vi "Get Feature Names.vi"(8 "error in (no error)":errorcluster caption="entrée d'erreur (pas d'erreur)", 9 "doc":string, 10 "X":string[][](array[string]), 11 "TfidfVectorizer.lvclass":refnum<class "TfidfVectorizer.lvclass">) -> (0 "error out":errorcluster caption="sortie d'erreur", 2 "Data":T1, 3 "TfidfVectorizer.lvclass":refnum<class "TfidfVectorizer.lvclass">)   [LabVIEW 2020, in "TfidfVectorizer.lvclass"]
doc: "Array mapping from feature integer indices to feature name.\n\nReturns : \n\n- feature_names : list\nA list of feature names."
uses:
  TfidfVectorizer.lvclass
  TfidfVectorizer.lvclass/TfidfVectorizer.ctl
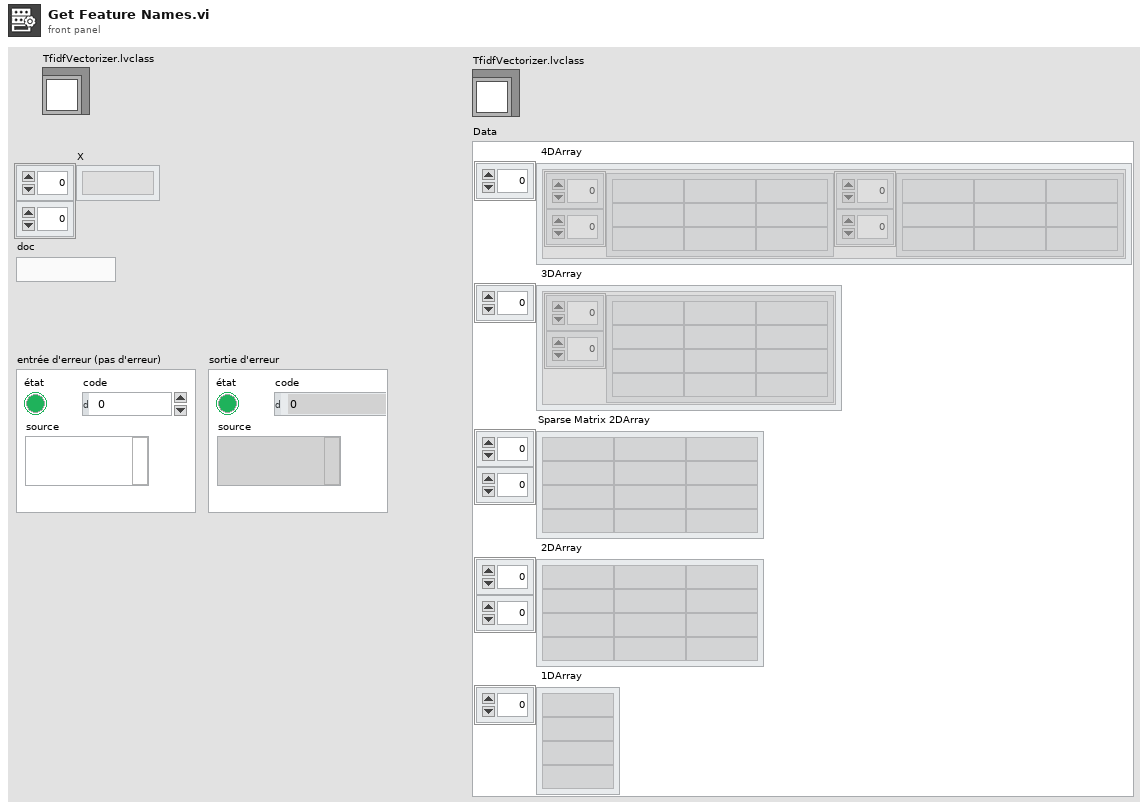
[diagram p1: front panel]
types:
  T1 = cluster{" 4DArray":cluster{"1":string[][], "2":string[][]}[], " 3DArray":cluster{"Tableau":string[][]}[], "Sparse Matrix 2DArray":string[][], " 2DArray":string[][], " 1DArray":string[]}
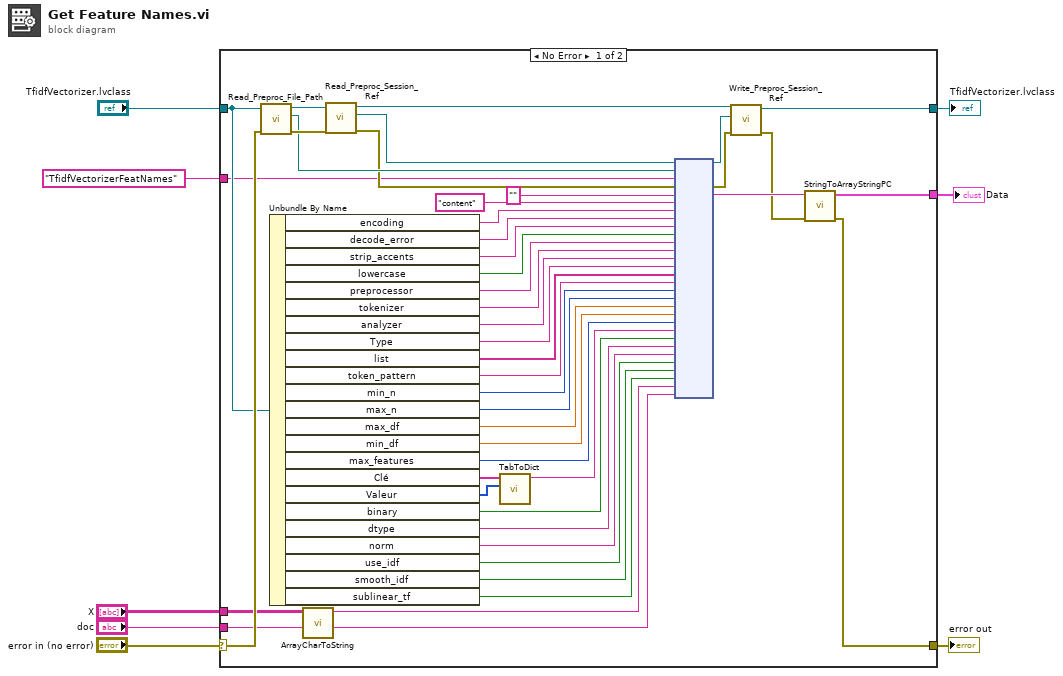
[diagram p0: block diagram]
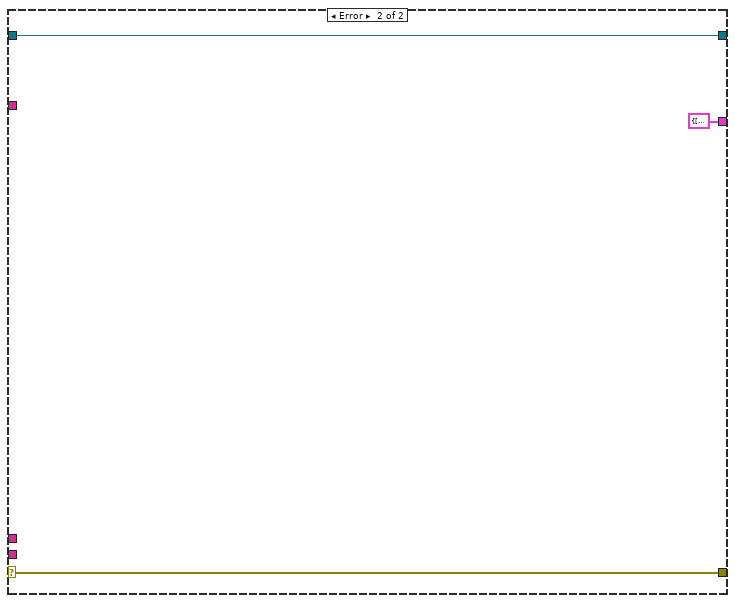
[diagram p2: hidden frame]
diagram:
  n1 = case shown="No Error" "error in (no error)" {
    selector: "error in (no error)" -> [w42 w56]
    tunnel: [w11 w56] -> w7
    tunnel: [w9 w55] -> w5
    tunnel: "TfidfVectorizer.lvclass" -> [w41 w55]
    tunnel: "TfidfVectorizerFeatNames" ("Fonction") -> [w40 _]
    tunnel: [w10 T1 {" 4DArray"=[], " 3DArray"=[], "Sparse Matrix 2DArray"=[], " 2DArray"=[], " 1DArray"=[]} ("Data")] -> w1
    tunnel: "X" -> [w15 _]
    tunnel: "doc" -> [w16 _]
    frame No Error {
      n2 = call-dynamic "Read_Preproc_File_Path.vi"("error in (no error)"=w42, "Python in"=w41) -> ("error out"=w52:errorcluster, "File_Path"=w51:path, "Python out"=w53:refnum<class "TfidfVectorizer.lvclass">)  [unwired: 7 in]
      n3 = Unbundle By Name(w41) -> ("encoding"=w44:string, "decode_error"=w43:string, "strip_accents"=w39:string, "lowercase"=w38:bool, "preprocessor"=w37:string, "tokenizer"=w36:string, "analyzer"=w35:string, "Type"=w33:string, "list"=w32:string[], "token_pattern"=w31:string, "min_n"=w30:i32, "max_n"=w29:i32, "max_df"=w28:dbl, "min_df"=w27:dbl, "max_features"=w26:i32, "Clé"=w25:string[], "Valeur"=w24:i32[], "binary"=w22:bool, "dtype"=w21:string, "norm"=w20:string, "use_idf"=w19:bool, "smooth_idf"=w18:bool, "sublinear_tf"=w17:bool)
      n4 = call "ArrayCharToString.vi"("TAB"=w15) -> ("Instruction"=w14:string)  [unwired: 10 in]
      n5 = call-dynamic "Read_Preproc_Session_Ref.vi"("error in (no error)"=w52, "Python in"=w53) -> ("error out"=w49:errorcluster, "Session_ref"=w50:refnum<k35>, "Python out"=w48:refnum<class "TfidfVectorizer.lvclass">)  [unwired: 7 in]
      n6 = call "TabToDict.vi"("Int Value"=w24, "String key"=w25) -> ("Dict with int value"=w23:string)  [unwired: 8 in, 1 out]
      n7 = node(w50, w51, w40, w49, "", "content", w44, w43, w39, w38, w37, w36, w35, w33, w32, w31, w30, w29, w28, w27, w26, w23, w22, w21, w20, w19, w18, w17, w14, w16) -> (w46:refnum<k35>, w47:errorcluster, w13:string)  [unwired: 25 in, 2 out]
      n8 = call-dynamic "Write_Preproc_Session_Ref.vi"("error in (no error)"=w47, "Session_ref"=w46, "Python in"=w48) -> ("error out"=w12:errorcluster, "Python out"=w9:refnum<class "TfidfVectorizer.lvclass">)  [unwired: 7 in]
      n9 = call "StringToArrayStringPC.vi"("sortie d'erreur"=w12, "Return value"=w13) -> ("sortie d'erreur"=w11:errorcluster, "Data"=w10:T1)  [unwired: 8 in]
    }
    frame Error {
    }
  }
  "error out" <- w7
  "TfidfVectorizer.lvclass" <- w5
  "Data" <- w1
